vi "process.vi"(8 "error in (no error)":errorcluster, 11 "MQTT_Base in":refnum<class "MQTT_Base.lvclass">) -> (0 "error out":errorcluster)   [LabVIEW 2013, in "MQTT Base.lvlib" / "MQTT_Base.lvclass"]
uses:
  MQTT_Base.lvclass
  MQTT_Base.lvclass/MQTT_Base.ctl
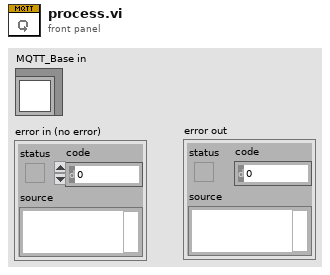
[diagram p1: front panel]
types:
  T1 = typedef "MQTT Base.lvlib/MQTT_Base.lvclass/Response -- cluster.ctl" = cluster{"Packet":refnum<class "ControlPacket.lvclass">, "Protocol Error":errorcluster, "disconnect session":bool, "[ACK]":refnum<notifier>[]}
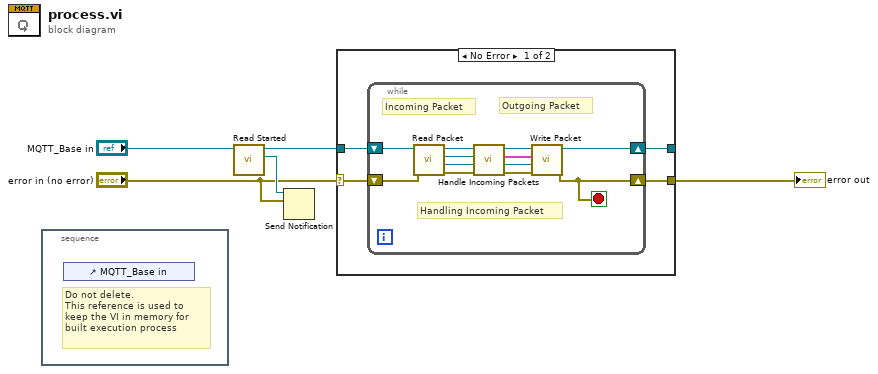
[diagram p0: block diagram]
diagram:
  n1 = stacked-sequence {
    frame #0 {
      # "Do not delete.\nThis reference is used to keep the VI in memory for built execution process"
      n2 = control-ref of="MQTT_Base in"() -> ()  [unwired: 1 out]
    }
  }
  n3 = call "Read Started.vi"("MQTT_Base in"="MQTT_Base in") -> ("Started"=w5:refnum<notifier>, "MQTT_Base out"=w3:refnum<class "MQTT_Base.lvclass">)  [unwired: 8 in, 1 out]
  n4 = Send Notification(notification="error in (no error)", notifier=w5) -> ()  [unwired: 1 in, 2 out]
  n5 = case shown="No Error" "error in (no error)" {
    selector: "error in (no error)" -> [w7 w23]
    tunnel: [w9 w23] -> w1
    tunnel: [w8 w22] -> _
    tunnel: w3 -> [w6 w22]
    frame No Error {
      n6 = while {
        shift-right: [w18] -> w8
        shift-left: w6 -> [w21]
        shift-right: [w10] -> w9
        shift-left: w7 -> [w11]
        stop <- w10 stop-if-true
        # "Handling Incoming Packet"
        # "Outgoing Packet"
        # "Incoming Packet"
        n7 = call "Read Packet.vi"("error in (no error)"=w11, "MQTT_Base in"=w21) -> ("error out"=w12:errorcluster, "SessionMailbox"=w14:refnum<queue>, "Packet"=w15:refnum<class "ControlPacket.lvclass">, "MQTT_Base out"=w20:refnum<class "MQTT_Base.lvclass">)  [unwired: 6 in]
        n8 = call-dynamic "Handle Incoming Packets.vi"("error in (no error)"=w12, "SessionMailbox"=w14, "Incoming Packet"=w15, "MQTT_Base in"=w20) -> ("error out"=w17:errorcluster, "SessionMailbox out"=w13:refnum<queue>, "Outgoing"=w16:T1, "MQTT_Base out"=w19:refnum<class "MQTT_Base.lvclass">)  [unwired: 4 in]
        n9 = call "Write Packet.vi"("error in (no error)"=w17, "SessionMailbox in"=w13, "Outgoing"=w16, "MQTT_Base in"=w19) -> ("error out"=w10:errorcluster, "MQTT_Base out"=w18:refnum<class "MQTT_Base.lvclass">)  [unwired: 6 in]
      }
    }
    frame Error {
    }
  }
  "error out" <- w1
